vi "Init Events.vi"(8 "error in (no error)":errorcluster, 11 "GUI Helper in":refnum<class "GUI Helper.lvclass">) -> (0 "error out":errorcluster, 3 "GUI Helper out":refnum<class "GUI Helper.lvclass">)   [LabVIEW 2020, in "VolatusGUI.lvlib" / "GUI Helper.lvclass"]
uses:
  GUI Helper.lvclass
  GUI Helper.lvclass/GUI Helper.ctl
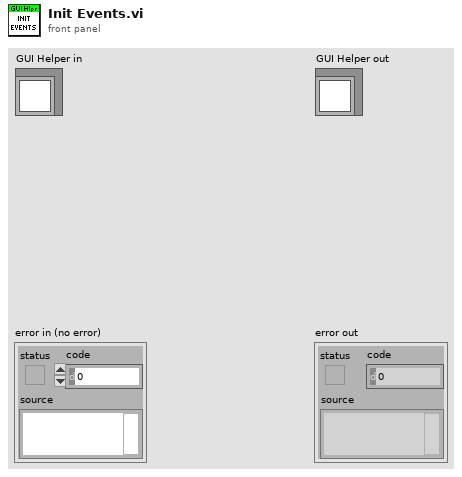
[diagram p1: front panel]
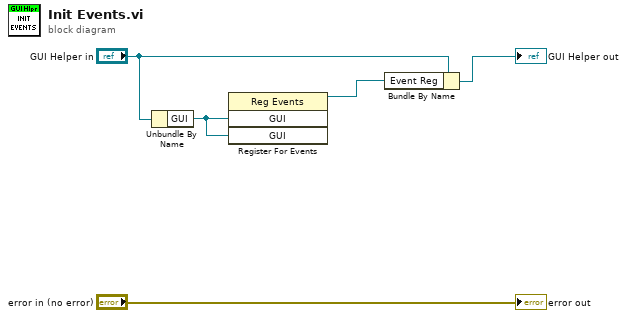
[diagram p0: block diagram]
diagram:
  n1 = Unbundle By Name("GUI Helper in") -> ("GUI"=w2:refnum<vi>)
  n2 = register-events(w2, w2) -> (reference out=w1:refnum<event-registration>)  [unwired: 2 in, 1 out]
  n3 = Bundle By Name(cluster="GUI Helper in", "Event Reg"=w1) -> (→"GUI Helper out":refnum<class "GUI Helper.lvclass">)
  "error out" <- "error in (no error)"
